vi "imaq_to_1d_array.vi"(8 "Error in":errorcluster caption="Error in (no error)", 11 "Image (in)":T1) -> (0 "Error out":errorcluster, 1 "Height":i32, 2 "Width":i32, 3 "Hst Src Image array (out)":u8[](array[numeric]))   [LabVIEW 2018]
uses:
  <vilib>/vision/Image Controls.llb/IMAQ Image.ctl
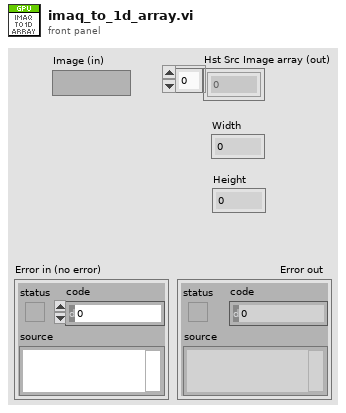
[diagram p1: front panel]
types:
  T1 = typedef "IMAQ Image.ctl" = refnum<image>
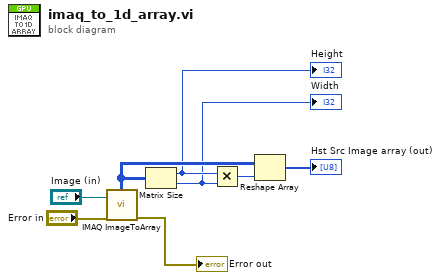
[diagram p0: block diagram]
diagram:
  n1 = call "IMAQ ImageToArray"("error in (no error)"="Error in", "Image"="Image (in)") -> ("error out"=→"Error out":errorcluster, "Image Pixels (U8)"=w8:u8[][])  [unwired: 2 in, 3 out]
  n2 = Matrix Size(0:w8) -> (1:w7:i32, 2:w6:i32)
  "Height" <- w7
  "Width" <- w6
  n3 = Multiply(x=w7, y=w6) -> (x*y=w1:i32)
  n4 = Reshape Array(w8, w1) -> (→"Hst Src Image array (out)":u8[])
